vi "DS345 SEND ARBWAVE ARRAYwithoffset.VI"(1 "y vertices / amplitude points":dbl[](array[numeric]) format="%.2f", 2 "x vertices for vector mode":i16[](array[numeric]) min=0 max=16299, 3 "error in":errorcluster, 4 "sampling FREQ.":sgl=40000000.0 min=0.002329 max=4e+07 format="%.6f", 5 "ARB.wave source":u16(ring) items=[".WAV file", "array in point mode", "array in vector mode"], 6 "GPIB address":string="19") -> (0 "error out":errorcluster)   [LabVIEW 2013]
doc: "This subVI is used to send data points of an arbitrary waveform to the DS345 . \n You can use LabVIEW functions to create arbitrary waveforms and connect the result to this subVI .\n Data can be sent in point mode or in vector mode .\n In point mode , data consists of amplitude points while in vector mode data is described as points with x- and y -vertices . \n If the function is set to ARBITRARY, the waveform will be output immediately ."
uses:
  <vilib>/Analysis/NI_AALBase.lvlib
panel:
  out "x/y":dbl format="%.2f"
  out "output string":string
  out "16bit integer":i16[](array[numeric])
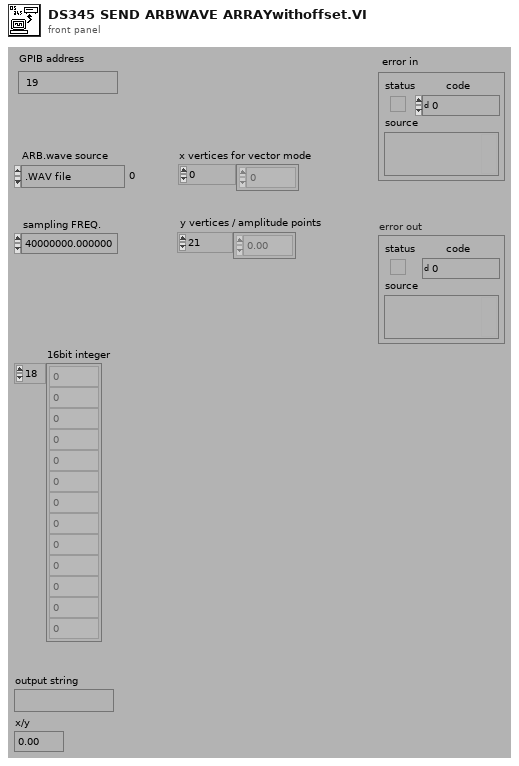
[diagram p1: front panel]
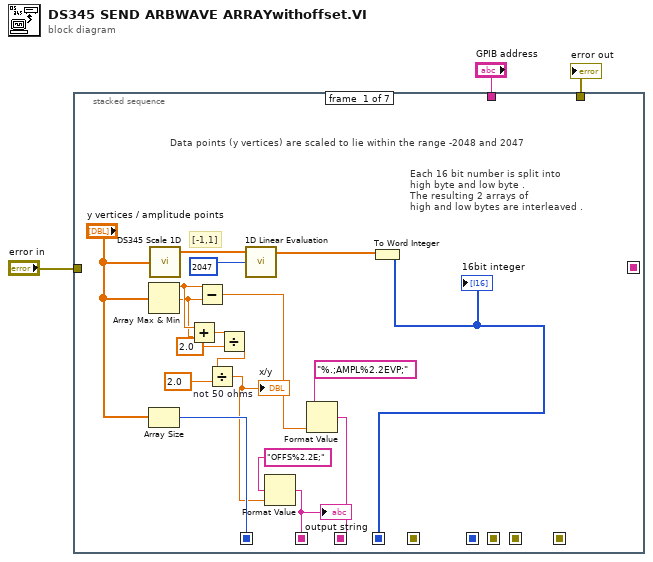
[diagram p0: block diagram]
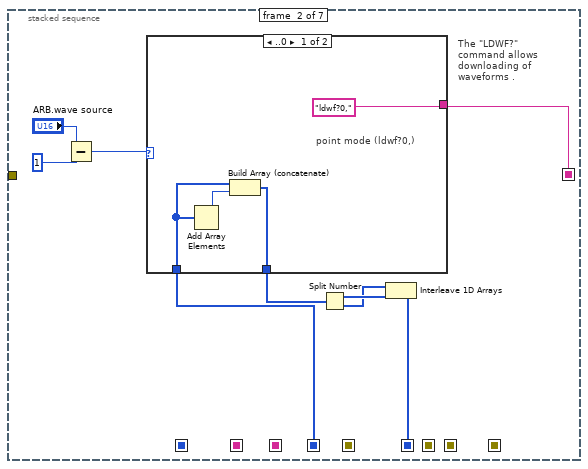
[diagram p2: hidden frame]
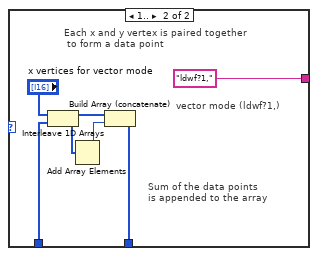
[diagram p3: hidden frame]
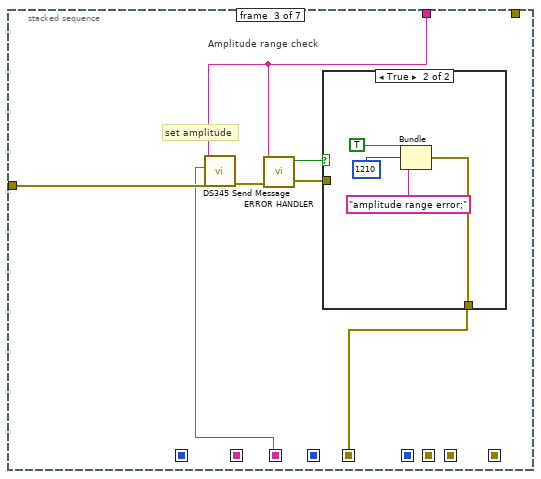
[diagram p4: hidden frame]
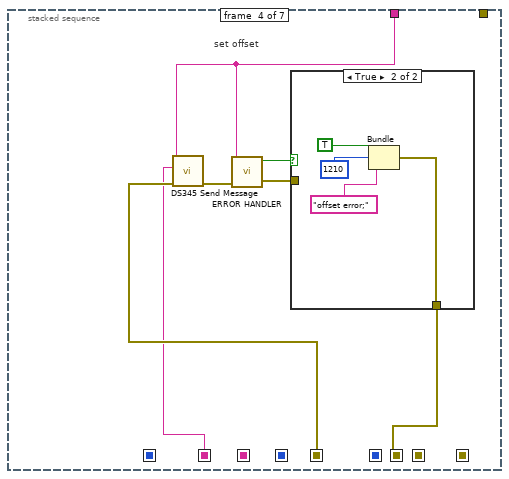
[diagram p6: hidden frame]
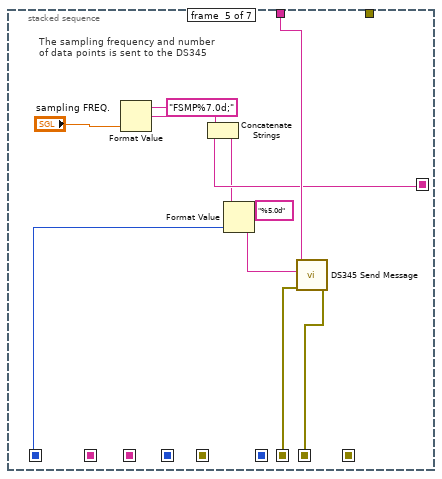
[diagram p8: hidden frame]
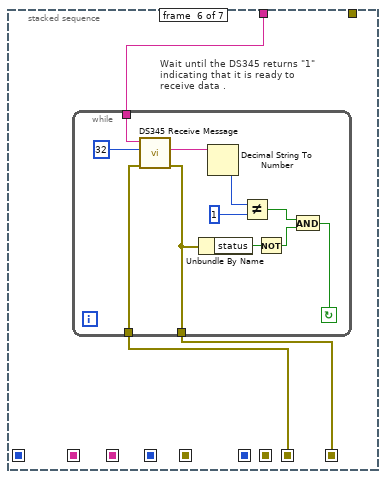
[diagram p9: hidden frame]
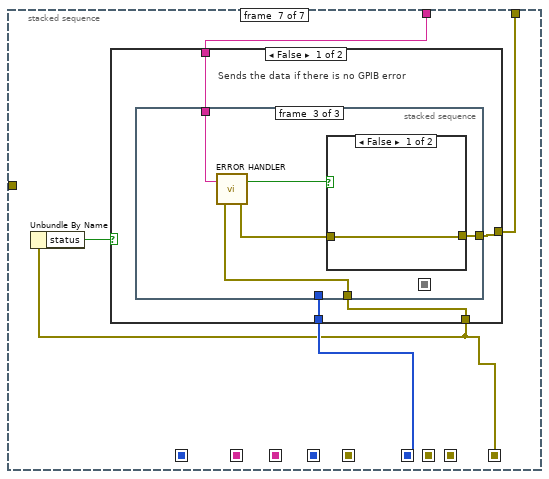
[diagram p10: hidden frame]
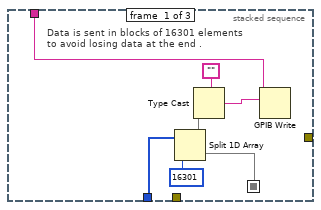
[diagram p11: hidden frame]
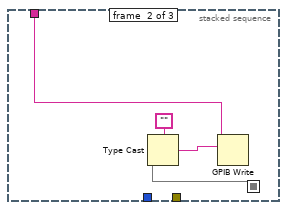
[diagram p12: hidden frame]
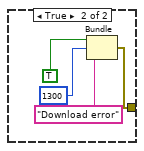
[diagram p13: hidden frame]
diagram:
  n1 = stacked-sequence {
    seq-local: [w16 _ _ _ _ _ _] -> [_ w28 _ _ _ _ _]
    seq-local: [_ _ _ _ _ w77 _] -> [_ _ _ _ _ _ w90]
    seq-local: [_ _ _ _ w72 _ _] -> [_ _ _ _ _ w76 _]
    seq-local: [w17 _ _ _ _ _ _] -> [_ _ w42 _ _ _ _]
    seq-local: [_ _ _ w54 _ _ _] -> [_ _ _ _ w65 _ _]
    seq-local: [w19 _ _ _ _ _ _] -> [_ _ _ _ w69 _ _]
    seq-local: [_ w24 _ _ _ _ _] -> [_ _ _ _ w67 _ _]
    seq-local: [_ w23 _ _ _ _ _] -> [_ _ _ _ _ _ w93]
    seq-local: [w11 _ _ _ _ _ _] -> [_ _ _ w53 _ _ _]
    seq-local: [_ _ w41 _ _ _ _] -> [_ _ _ w55 _ _ _]
    tunnel: "GPIB address" -> [_ _ w43 w56 w71 w78 w94]
    tunnel: "error in" -> [_ _ w44 _ _ _ _]
    tunnel: [_ _ _ _ _ _ w92] -> w1
    frame #0 {
      # "[-1,1]"
      # "Each 16 bit number is split into \nhigh byte and low byte .\nThe resulting 2 arrays of \nhigh and low bytes are interleaved ."
      # "Data points (y vertices) are scaled to lie within the range -2048 and 2047"
      n2 = Array Max & Min(array="y vertices / amplitude points") -> (max value=w10:dbl, min value=w9:dbl)  [unwired: 2 out]
      n3 = Array Size(array="y vertices / amplitude points") -> (size(s)=w19:i32)
      n4 = call "DS345 Scale 1D.vi"("X"="y vertices / amplitude points") -> ("Y=(X-offset)/scale"=w21:dbl[])  [unwired: 3 out]
      n5 = Add(x=w10, y=w9) -> (x+y=w8:dbl)
      n6 = Subtract(x=w10, y=w9) -> (x-y=w13:dbl)
      n7 = Divide(x=w8, y=2.0) -> (x/y=w5:dbl)
      n8 = Divide "not 50 ohms"(x=w5, y=2.0) -> (x/y=w4:dbl)
      "x/y" <- w4
      n9 = call <vilib>:"1D Linear Evaluation.vi"("scale"=2047, "X"=w21) -> ("Y[i]=X[i]*a+b"=w14:dbl[])  [unwired: 1 in, 1 out]
      n10 = Format Value(format string="OFFS%2.2E;", value (0)=w4) -> (output string=w11:string)  [unwired: 1 in]
      "output string" <- w11
      n11 = Format Value(format string="%.;AMPL%2.2EVP;", value (0)=w13) -> (output string=w17:string)  [unwired: 1 in]
      n12 = To Word Integer(number=w14) -> (16bit integer=w16:i16[])
      "16bit integer" <- w16
    }
    frame #1 {
      # "The \"LDWF?\" \ncommand allows \ndownloading of\nwaveforms ."
      n13 = Subtract(x="ARB.wave source", y=1) -> (x-y=w29:i32)
      n14 = case shown="..0" w29 {
        tunnel: w28 -> [w34 w40]
        tunnel: [w32 w37] -> w25
        tunnel: ["ldwf?0," "ldwf?1,"] -> w24
        frame ..0 {
          # "point mode (ldwf?0,)"
          n15 = Add Array Elements(numeric array=w34) -> (sum=w33:i16)
          n16 = Build Array (concatenate)(w34, w33) -> (w32:i16[])
        }
        frame 1.. {
          # "vector mode (ldwf?1,)"
          # "Sum of the data points\nis appended to the array"
          # "Each x and y vertex is paired together\n to form a data point"
          n17 = Interleave 1D Arrays("x vertices for vector mode", w40) -> (w39:i16[])
          n18 = Add Array Elements(numeric array=w39) -> (sum=w38:i16)
          n19 = Build Array (concatenate)(w39, w38) -> (w37:i16[])
        }
      }
      n20 = Split Number(x=w25) -> (hi(x)=w27:u8[], lo(x)=w26:u8[])
      n21 = Interleave 1D Arrays(w26, w27) -> (w23:u8[])
    }
    frame #2 {
      # "set amplitude"
      # "Amplitude range check"
      n22 = call "DS345 Send Message.vi"("address string"=w43, "write buffer"=w42, "error in"=w44) -> ("error out"=w47:errorcluster)  [unwired: 3 in, 3 out]
      n23 = call "ERROR HANDLER.vi"("error in"=w47, "GPIB address"=w43) -> ("error out"=w45:errorcluster, "error found"=w46:bool)
      n24 = case shown="True" w46 {
        tunnel: [w48 w49] -> w41
        tunnel: w45 -> [w48 _]
        frame False {
        }
        frame True {
          n25 = Bundle(TRUE, 1210, "amplitude range error;") -> (w49:errorcluster)  [unwired: 1 in]
        }
      }
    }
    frame #3 {
      # "set offset"
      n26 = call "DS345 Send Message.vi"("address string"=w56, "write buffer"=w53, "error in"=w55) -> ("error out"=w59:errorcluster)  [unwired: 3 in, 3 out]
      n27 = call "ERROR HANDLER.vi"("error in"=w59, "GPIB address"=w56) -> ("error out"=w57:errorcluster, "error found"=w58:bool)
      n28 = case shown="True" w58 {
        tunnel: [w60 w61] -> w54
        tunnel: w57 -> [w60 _]
        frame False {
        }
        frame True {
          n29 = Bundle(TRUE, 1210, "offset error;") -> (w61:errorcluster)  [unwired: 1 in]
        }
      }
    }
    frame #4 {
      # "The sampling frequency and number\nof data points is sent to the DS345"
      n30 = Format Value(format string="FSMP%7.0d;", value (0)="sampling FREQ.") -> (output string=w68:string)  [unwired: 1 in]
      n31 = Concatenate Strings(w68, w67) -> (w66:string)
      n32 = Format Value(string ("")=w66, format string="%5.0d", value (0)=w69) -> (output string=w73:string)
      n33 = call "DS345 Send Message.vi"("address string"=w71, "write buffer"=w73, "error in"=w65) -> ("error out"=w72:errorcluster)  [unwired: 3 in, 3 out]
    }
    frame #5 {
      # "Wait until the DS345 returns \"1\" \nindicating that it is ready to\nreceive data ."
      n34 = while {
        tunnel: w78 -> [w85]
        tunnel: [w80] -> w77
        tunnel: w76 -> [w86]
        stop <- w82 continue-if-true
        n35 = call "DS345 Receive Message.vi"("address string"=w85, "byte count"=32, "error in"=w86) -> ("read buffer"=w81:string, "error out"=w80:errorcluster)  [unwired: 3 in, 2 out]
        n36 = Unbundle By Name(w80) -> ("status"=w79:bool)
        n37 = Decimal String To Number(string=w81) -> (number=w88:i32)  [unwired: 2 in, 1 out]
        n38 = Not Equal?(x=w88, y=1) -> (x != y?=w84:bool)
        n39 = Not(x=w79) -> (.not. x?=w83:bool)
        n40 = And(x=w84, y=w83) -> (x .and. y?=w82:bool)
      }
    }
    frame #6 {
      n41 = Unbundle By Name(w90) -> ("status"=w91:bool)
      n42 = case shown="False" w91 {
        tunnel: w93 -> [w98 _]
        tunnel: w94 -> [w97 _]
        tunnel: [w96 w120] -> w92
        tunnel: w90 -> [w95 w120]
        frame False {
          # "Sends the data if there is no GPIB error"
          n43 = stacked-sequence {
            seq-local: [w101 _ _] -> [_ w106 _]
            tunnel: w98 -> [w100 _ _]
            tunnel: w97 -> [w99 w107 w113]
            tunnel: [_ _ w114] -> w96
            tunnel: w95 -> [_ _ w112]
            frame #0 {
              # "Data is sent in blocks of 16301 elements\nto avoid losing data at the end ."
              n44 = Split 1D Array(array=w100, index=16301) -> (first subarray=w103:u8[], second subarray=w101:u8[])
              n45 = Type Cast(type="", x=w103) -> (*(type *) &x=w104:string)
              n46 = GPIB Write(0:w99, 1:w104) -> ()  [unwired: 3 in, 2 out]
            }
            frame #1 {
              n47 = Type Cast(type="", x=w106) -> (*(type *) &x=w108:string)
              n48 = GPIB Write(0:w107, 1:w108) -> ()  [unwired: 3 in, 2 out]
            }
            frame #2 {
              n49 = call "ERROR HANDLER.vi"("error in"=w112, "GPIB address"=w113) -> ("error out"=w111:errorcluster, "error found"=w110:bool)
              n50 = case shown="False" w110 {
                tunnel: [w115 w116] -> w114
                tunnel: w111 -> [w115 _]
                frame False {
                }
                frame True {
                  n51 = Bundle(TRUE, 1300, "Download error") -> (w116:errorcluster)  [unwired: 1 in]
                }
              }
            }
          }
        }
        frame True {
        }
      }
    }
  }
  "error out" <- w1
